vi "ExecuteSkill.vi"(0 "object in":refnum<class "AlignToKick.lvclass">, 2 "Robot in":refnum<class "Robot.lvclass">, 4 "GameRef":refnum<data-value>, 5 "error in (no error)":errorcluster) -> (14 "object out":refnum<class "AlignToKick.lvclass">, 16 "Robot out":refnum<class "Robot.lvclass">, 19 "error out":errorcluster)   [LabVIEW 2023, in "AlignToKick.lvclass"]
uses:
  AlignToKick.lvclass
  C:/Users/ebert/Documents/codes/SSL/repo/SSL_AI/AlignSkill/AlignSkill.lvclass
  Robot_class/Robot.lvclass
  Game_class/Game.lvclass
  Robot_class/Robot.lvclass/Robot.ctl
  Game_class/Game.lvclass/Game.ctl
  Object_class/Object.lvclass/Object.ctl
  Game_class/Read BallRef.vi
  Object_class/Read position(x,y).vi
  Robot_class/Read dest_x_kick.vi
  Robot_class/Read dest_y_kick.vi
  Ball_class/Ball.lvclass
  C:/Users/ebert/Documents/codes/SSL/repo/SSL_AI/Object_class/Object.lvclass
  AlignSkill/AlignSkill.lvclass
panel:
  in  "normFactor":dbl
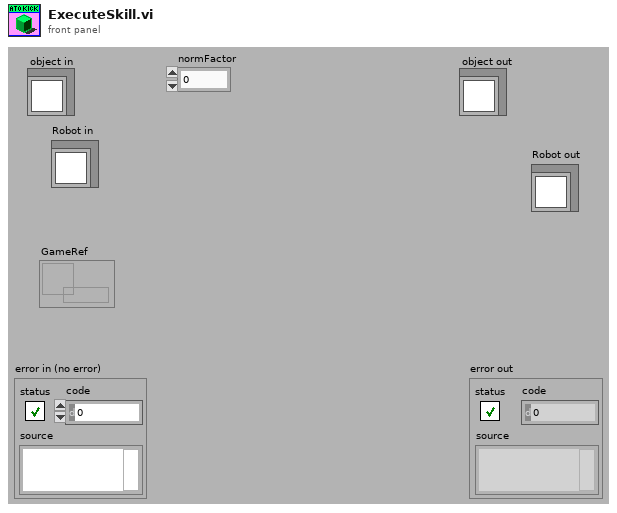
[diagram p1: front panel]
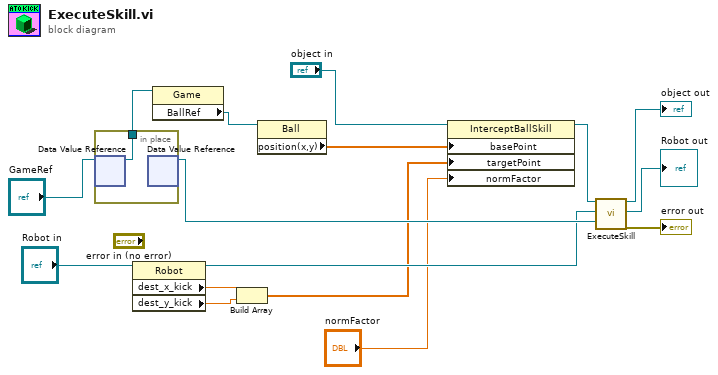
[diagram p0: block diagram]
diagram:
  n1 = in-place {
    in-place-border: [w17] -> w12
    n2 = in-place-dvr #1("GameRef") -> (w17:refnum<class "Game.lvclass">)  [unwired: 1 out]
    n3 = in-place-dvr #1() -> (w4:refnum<data-value>)  [unwired: 1 in, 1 out]
  }
  n4 = property class="Robot"(reference="Robot in") -> (reference out=w3:refnum<class "Robot.lvclass">, "dest_x_kick"=w7:dbl, "dest_y_kick"=w6:dbl)  [unwired: 1 in, 1 out]
  n5 = property class="Game"(reference=w12) -> ("BallRef"=w11:refnum<class "Ball.lvclass">)  [unwired: 1 in, 2 out]
  n6 = Build Array(w7, w6) -> (w2:dbl[])
  n7 = property class="Ball"(reference=w11) -> ("position(x,y)"=w10:dbl[])  [unwired: 1 in, 2 out]
  n8 = property class="InterceptBallSkill"(reference="object in", "basePoint"=w10, "targetPoint"=w2, "normFactor"="normFactor") -> (reference out=w9:refnum<class "AlignToKick.lvclass">)  [unwired: 1 in, 1 out]
  n9 = call-parent "ExecuteSkill.vi"("object in"=w9, "Robot in"=w3, "GameRef"=w4) -> ("object out"=→"object out":refnum<class "AlignToKick.lvclass">, "Robot out"=→"Robot out":refnum<class "Robot.lvclass">, "error out"=→"error out":errorcluster)  [unwired: 14 in]
